vi "配置文件保存.vi"   [LabVIEW 2016, in "斯坦道CODMn.lvlib"]
uses:
  <vilib>/Utility/config.llb/NI_LVConfig.lvlib
types:
  T1 = typedef "NI_LVConfig.lvlib/Config Data RefNum.ctl" = refnum<k1>
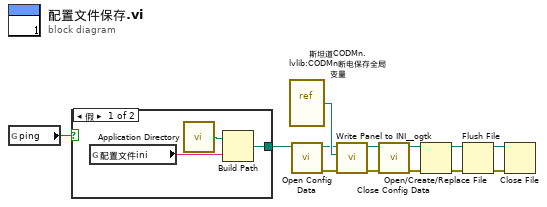
[diagram p0: block diagram]
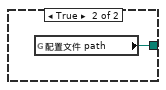
[diagram p2: hidden frame]
diagram:
  n1 = global read "CODMN外部API.vi" "ping"() -> (w12:bool)
  n2 = case shown="假" w12 {
    tunnel: [w14 w17] -> w13
    frame False {
      n3 = global read "COD内部交互全局.vi" "配置文件ini"() -> (w16:string)
      n4 = call <vilib>:"Application Directory.vi"() -> ("Application Directory"=w15:path)
      n5 = Build Path(base path=w15, name or relative path=w16) -> (appended path=w14:path)
    }
    frame True {
      n6 = global read "CODMN外部API.vi" "配置文件 path"() -> (w17:path)
    }
  }
  n7 = vi-ref "斯坦道CODMn.lvlib:CODMn断电保存全局变量.vi"() -> (w2:refnum<vi>)
  n8 = call <vilib>:"Open Config Data.vi"("configuration file path"=w13) -> ("error out"=w4:errorcluster, "refnum"=w1:T1)  [unwired: 8 in, 1 out]
  n9 = call <userlib>:"Write Panel to INI__ogtk.vi"("error in (no error)"=w4, "VI ref"=w2, "refnum"=w1) -> ("error out"=w5:errorcluster, "refnum out"=w3:T1)  [unwired: 7 in]
  n10 = call <vilib>:"Close Config Data.vi"("error in (no error)"=w5, "refnum"=w3) -> ("error out"=w10:errorcluster, "file path"=w11:path)  [unwired: 8 in]
  n11 = Open/Create/Replace File(file path (use dialog)=w11, error in=w10) -> (refnum out=w7:refnum<file>, error out=w6:errorcluster)  [unwired: 4 in, 1 out]
  n12 = Flush File(refnum=w7, error in=w6) -> (refnum out=w8:refnum<file>, error out=w9:errorcluster)
  n13 = Close File(refnum=w8, error in=w9) -> ()  [unwired: 2 out]
